vi "Write Valve Position.vi"(8 "error in (no error)":errorcluster, 10 "Valve Position":refnum<vi>, 11 "Valve in":refnum<class "Valve.lvclass">) -> (0 "error out":errorcluster, 3 "Valve out":refnum<class "Valve.lvclass">)   [LabVIEW 2013, in "Valve.lvlib" / "Valve.lvclass"]
uses:
  Valve.lvclass
  Valve.lvclass/Valve.ctl
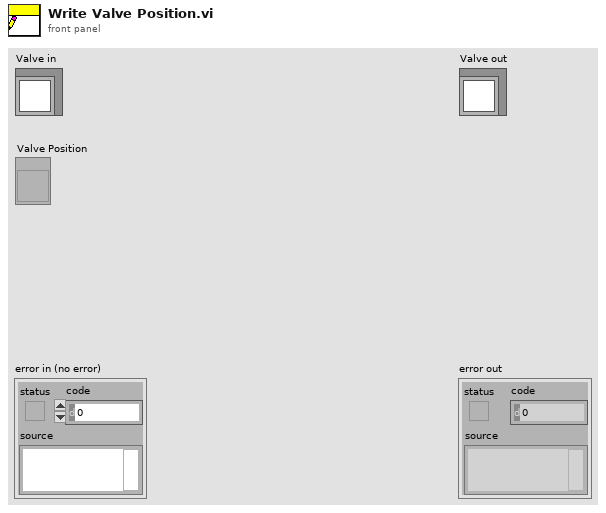
[diagram p1: front panel]
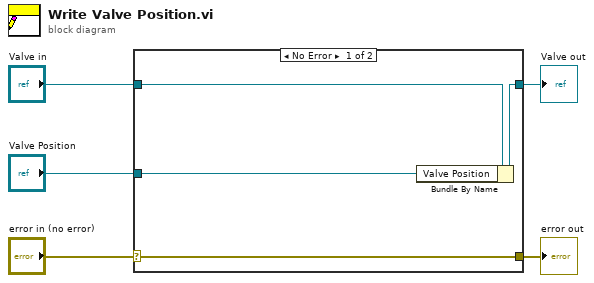
[diagram p0: block diagram]
diagram:
  n1 = case shown="No Error" "error in (no error)" {
    selector: "error in (no error)" -> [w9 w10]
    tunnel: [w9 w10] -> w4
    tunnel: [w7 w11] -> w2
    tunnel: "Valve in" -> [w8 w11]
    tunnel: "Valve Position" -> [w6 _]
    frame No Error {
      n2 = Bundle By Name(cluster=w8, "Valve Position"=w6) -> (w7:refnum<class "Valve.lvclass">)
    }
    frame Error {
    }
  }
  "error out" <- w4
  "Valve out" <- w2
